vi "Get Private Global Path.vi"() -> (3 "appended path":path)   [LabVIEW 2016]
uses:
  Constants/Public/Get Constants.vi
  Constants/Constants.lvlib
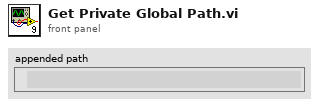
[diagram p1: front panel]
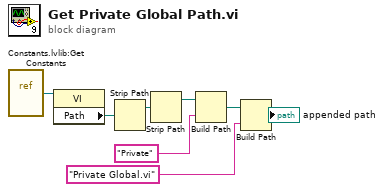
[diagram p0: block diagram]
diagram:
  n1 = vi-ref "Constants.lvlib:Get Constants.vi"() -> (w1:refnum<vi>)
  n2 = property class="VI"(reference=w1) -> ("Path"=w2:path)  [unwired: 1 in, 2 out]
  n3 = Strip Path(path=w2) -> (stripped path=w3:path)  [unwired: 1 out]
  n4 = Strip Path(path=w3) -> (stripped path=w4:path)  [unwired: 1 out]
  n5 = Build Path(base path=w4, name or relative path="Private") -> (appended path=w6:path)
  n6 = Build Path(base path=w6, name or relative path="Private Global.vi") -> (appended path=→"appended path":path)
